vi "Gen 2D objects.vi"() -> ()   [LabVIEW 2019]
uses:
  <vilib>/picture/picture.llb/imagedata.ctl
panel:
  out "image data":T1
  out "new picture":picture
  in  "doodle":path=path "C:/Users/nitest/Downloads/Game/Game/monito1.png"
  in  "background":path=path "C:/Users/nitest/Documents/background.png"
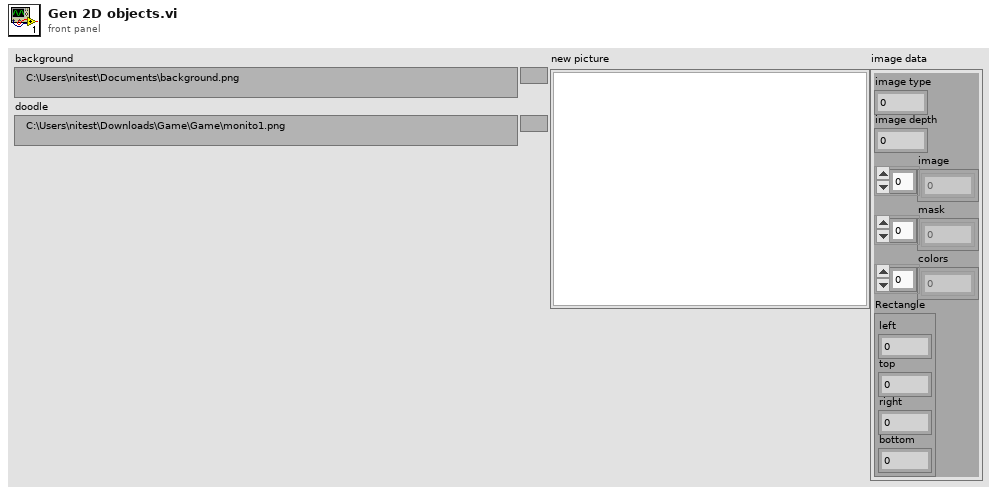
[diagram p1: front panel]
types:
  T1 = typedef "imagedata.ctl" = cluster{"image type":i32, "image depth":i32, "image":u8[], "mask":u8[], "colors":u32[], "Rectangle":cluster{"left":i16, "top":i16, "right":i16, "bottom":i16}}
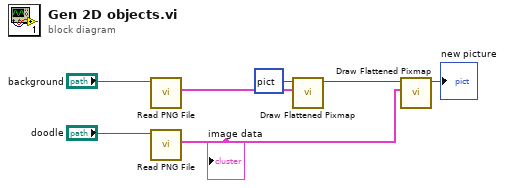
[diagram p0: block diagram]
diagram:
  n1 = call <vilib>:"Read PNG File.vi"("path to PNG file"="background") -> ("image data"=w5:T1)  [unwired: 8 in, 2 out]
  n2 = call <vilib>:"Read PNG File.vi"("path to PNG file"="doodle") -> ("image data"=w3:T1)  [unwired: 8 in, 2 out]
  "image data" <- w3
  n3 = call <vilib>:"Draw Flattened Pixmap.vi"("image data"=w5, "picture"=picture data[5B]) -> ("new picture"=w2:picture)  [unwired: 7 in]
  n4 = call <vilib>:"Draw Flattened Pixmap.vi"("image data"=w3, "picture"=w2) -> ("new picture"=→"new picture":picture)  [unwired: 7 in]
